vi "Global Trampa 0.vi"() -> ()   [LabVIEW 2019]
panel:
  out "Forza rif":bool
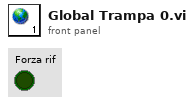
[diagram p1: front panel]
diagram:
